vi "XNET CAN Signal Logger.vi"() -> ()   [LabVIEW 2021, in "XNET-CAN-Signal-Logger.lvlib"]
uses:
  XNET-CAN-Signal-Logger.lvlib
  <vilib>/xnet/xnet.llb/XNET Create Session (Signal Input Waveform).vi
  <vilib>/xnet/xnet.llb/XNET Read (Signal Waveform) .vi
  <resource>/objmgr/xnet.rc
panel:
  out "stopped":bool
  out "data":waveform(dbl)[](array[waveform])
  out "Signal Units":string[](array[string])
  out "Signal Values":dbl[](array[numeric])
  in  "Signals to Monitor":string[](array[combo])
  out "#Signals":i32
  in  "Start":bool
  out "error out":errorcluster
  out "Parsed Log file name":string
  in  "Log file name":string="LogFile_{Year}-{Month}-{Day}-{Hour}-{Minute}-{Second}.tdms"
  in  "Log file folder":path=path "C:/Users/NI/Desktop/Data"
  in  "Sample Rate (Hz)":dbl=100.0 format="%#_13g"
  in  "CAN Interface":refnum<k21>="CAN1"
  in  "XNET Cluster":refnum<k21>="ManyXnetChannels"
  in  "stop":bool
  # "Configuration"
  # "Signals to Monitor"
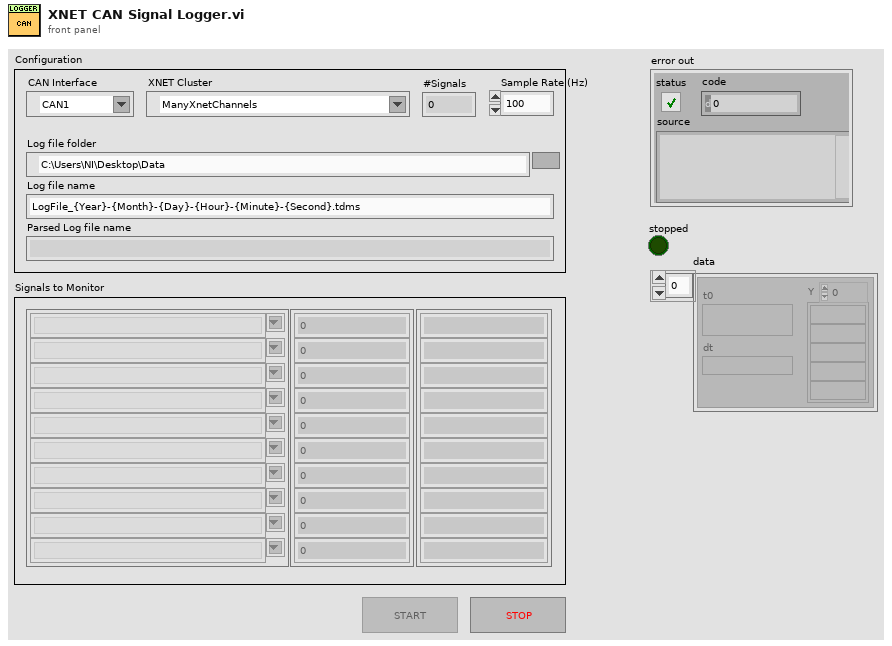
[diagram p1: front panel]
types:
  T1 = enum8{"Enabled", "Disabled", "Disabled and Grayed Out"}
  T2 = enum16{"open", "open or create", "create or replace", "create", "open (read-only)"}
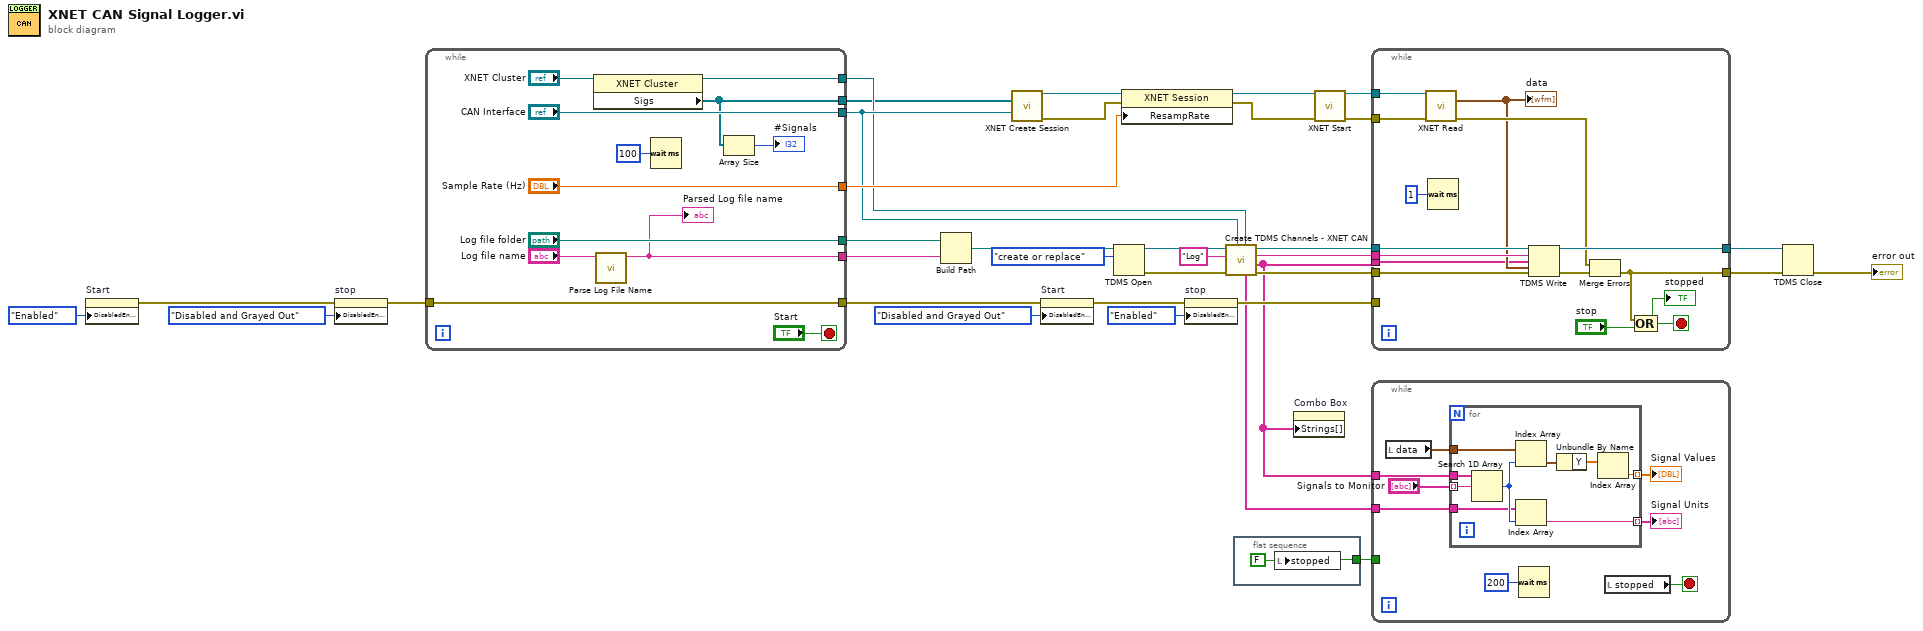
[diagram p0: block diagram]
diagram:
  n1 = property on="Start" class="Bool"("DisabledEnum"=T1."Enabled" ("Disabled")) -> (error out=w5:errorcluster)  [unwired: 2 in, 1 out]
  n2 = property on="stop" class="Bool"(error in=w5, "DisabledEnum"=T1."Disabled and Grayed Out" ("Disabled")) -> (error out=w12:errorcluster)  [unwired: 1 in, 1 out]
  n3 = while {
    tunnel: ["Sample Rate (Hz)"] -> w33
    tunnel: ["Log file folder"] -> w21
    tunnel: [w44] -> w19
    tunnel: ["CAN Interface"] -> w15
    tunnel: [w38] -> w14
    tunnel: w12 -> [w40]
    tunnel: [w40] -> w8
    tunnel: [w36] -> w4
    stop <- "Start" stop-if-true
    n4 = property class="XNET Cluster"(reference="XNET Cluster") -> (reference out=w38:refnum<k21>, "Sigs"=w36:refnum<k21>[])  [unwired: 1 in, 1 out]
    n5 = call "Parse Log File Name.vi"("Log file name"="Log file name") -> ("Parsed Log file name"=w44:string)  [unwired: 10 in]
    "Parsed Log file name" <- w44
    n6 = Wait (ms)(milliseconds to wait=u32 100) -> ()  [unwired: 1 out]
    n7 = Array Size(array=w36) -> (size(s)=→"#Signals":i32)
  }
  n8 = Build Path(base path=w21, name or relative path=w19) -> (appended path=w22:path)
  n9 = call-poly <vilib>:"XNET Create Session.vi"("signal list"=w4, "interface"=w15) -> ("session out"=w35:refnum<k21>, "error out"=w34:errorcluster)  [unwired: 12 in]
  n10 = property on="Start" class="Bool"(error in=w8, "DisabledEnum"=T1."Disabled and Grayed Out" ("Disabled")) -> (error out=w7:errorcluster)  [unwired: 1 in, 1 out]
  n11 = TDMS Open(10:T2."create or replace" ("operation (0:open)"), 11:w22) -> (0:w25:errorcluster, 3:w27:refnum<k34>)  [unwired: 5 in]
  n12 = property class="XNET Session"(reference=w35, error in=w34, "ResampRate"=w33) -> (reference out=w32:refnum<k21>, error out=w31:errorcluster)
  n13 = property on="stop" class="Bool"(error in=w7, "DisabledEnum"=T1."Enabled" ("Disabled")) -> (error out=w10:errorcluster)  [unwired: 1 in, 1 out]
  n14 = call "Create TDMS Channels - XNET CAN.vi"("XNET Cluster"=w14, "CAN Interface"=w15, "error in (no error)"=w25, "group name in"="Log", "TDMS ref in"=w27) -> ("error out"=w24:errorcluster, "Signal Names"=w3:string[], "group name out"=w20:string, "TDMS ref out"=w26:refnum<k34>, "Signal Units"=w2:string[])  [unwired: 2 in]
  n15 = flat-sequence {
    tunnel: [w48] -> w1
    frame #0 {
      w48 = FALSE ("stopped")
      n16 = local write "stopped"(w48) -> ()
    }
  }
  n17 = property on="Combo Box" class="CmbBox"("Strings[]"=w3) -> ()  [unwired: 2 in, 2 out]
  n18 = call <vilib>:"XNET Start.vi"("session in"=w32, "error in (no error)"=w31) -> ("session out"=w29:refnum<k21>, "error out"=w30:errorcluster)  [unwired: 12 in]
  n19 = while {
    tunnel: w29 -> [w62]
    tunnel: w30 -> [w61]
    tunnel: [w57] -> w28
    tunnel: w3 -> [w49]
    tunnel: w26 -> [w55]
    tunnel: w24 -> [w54]
    tunnel: w20 -> [w53]
    tunnel: [w51] -> w17
    tunnel: w10 -> [_]
    stop <- w59 stop-if-true
    n20 = call-poly <vilib>:"XNET Read.vi"("session in"=w62, "error in (no error)"=w61) -> ("data"=w50:waveform(dbl)[], "error out"=w52:errorcluster)  [unwired: 11 in, 1 out]
    "data" <- w50
    n21 = Wait (ms)(milliseconds to wait=u32 1) -> ()  [unwired: 1 out]
    n22 = TDMS Write(0:w55, 5:w53, 7:w49, 9:w50, 11:w54) -> (4:w57:refnum<k34>, 15:w56:errorcluster)  [unwired: 1 in, 2 out]
    n23 = Merge Errors(w52, w56) -> (w51:errorcluster)
    n24 = Compound Arithmetic op=OR(w51, "stop") -> (w59:bool)
    "stopped" <- w59
  }
  n25 = while {
    tunnel: w3 -> [w70]
    tunnel: w2 -> [w66]
    tunnel: w1 -> [_]
    stop <- w63 stop-if-true
    n26 = local read "data"() -> (w65:waveform(dbl)[])
    n27 = for {
      tunnel: "Signals to Monitor" -> [w79] mode=indexing
      tunnel: w70 -> [w78]
      tunnel: w65 -> [w77]
      tunnel: [w75] -> w68 mode=indexing
      tunnel: w66 -> [w72]
      tunnel: [w71] -> w69 mode=indexing
      n28 = Search 1D Array(1D array=w78, element=w79) -> (index of element=w73:i32)  [unwired: 1 in]
      n29 = Index Array(array=w77, index=w73) -> (element=w74:waveform(dbl))
      n30 = Index Array(array=w72, index=w73) -> (element=w71:string)
      n31 = Unbundle By Name(w74) -> ("Y"=w76:dbl[])
      n32 = Index Array(array=w76) -> (element=w75:dbl)  [unwired: 1 in]
    }
    "Signal Values" <- w68
    "Signal Units" <- w69
    n33 = Wait (ms)(milliseconds to wait=u32 200) -> ()  [unwired: 1 out]
    n34 = local read "stopped"() -> (w63:bool)
  }
  n35 = TDMS Close(8:w17, 11:w28) -> (0:→"error out":errorcluster)  [unwired: 1 out]
